vi "ReadPanelData.vi"(8 "error in (no error)":errorcluster, 11 "MAUI in":refnum<class "SMO.UI.MAUI.lvclass">) -> (0 "error out":errorcluster, 3 "MAUI out":refnum<class "SMO.UI.MAUI.lvclass">)   [LabVIEW 2019, in "SMO.UI.MAUI.lvclass"]
uses:
  SMO.UI.MAUI.lvclass
  Typedefs/PanelData.ctl
panel:
  in  "timeout in ms (-1)":i32
  out "last notification":T1[](array[typedef])
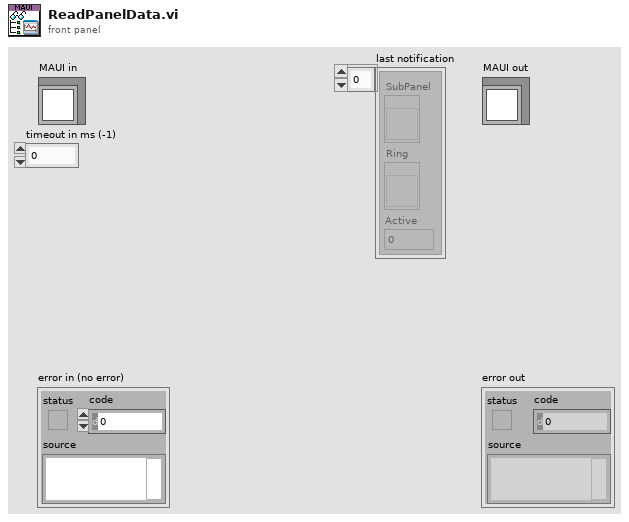
[diagram p1: front panel]
types:
  T1 = typedef "SMO.UI.MAUI.lvclass/PanelData.ctl" = cluster{"SubPanel":refnum<vi>, "Ring":refnum<vi>, "Active":i32}
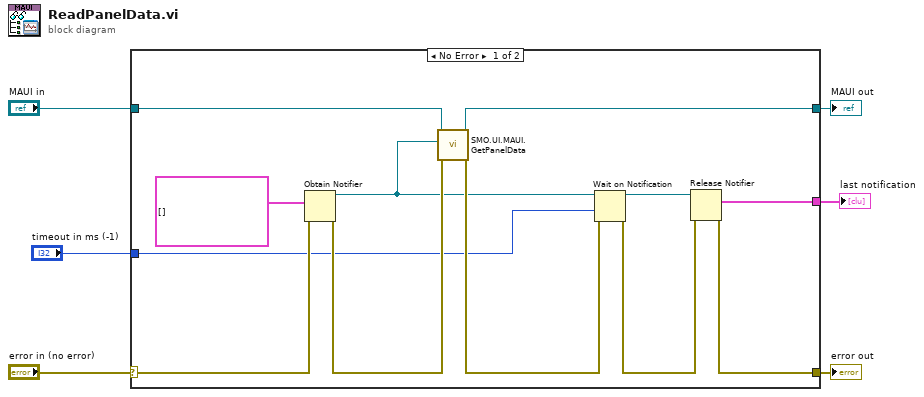
[diagram p0: block diagram]
diagram:
  n1 = case shown="No Error" "error in (no error)" {
    selector: "error in (no error)" -> [w18 w20]
    tunnel: [w14 w20] -> w5
    tunnel: [w8 w19] -> w3
    tunnel: "MAUI in" -> [w9 w19]
    tunnel: [w10 _] -> w2
    tunnel: "timeout in ms (-1)" -> [w7 _]
    frame No Error {
      n2 = Obtain Notifier(notification data type=T1[] [] ("Panel Data Array"), error in (no error)=w18) -> (notifier out=w11:refnum<notifier>, error out=w17:errorcluster)  [unwired: 2 in, 1 out]
      n3 = call "SMO.UI.MAUI.GetPanelData.vi"("error in (no error)"=w17, "GetPanelData"=w11, "MAUI"=w9) -> ("error out"=w16:errorcluster, "MAUI out"=w8:refnum<class "SMO.UI.MAUI.lvclass">)  [unwired: 7 in]
      n4 = Wait on Notification(notifier=w11, timeout in ms (-1)=w7, error in (no error)=w16) -> (notifier out=w12:refnum<notifier>, error out=w15:errorcluster)  [unwired: 1 in, 2 out]
      n5 = Release Notifier(notifier=w12, error in (no error)=w15) -> (last notification=w10:T1[], error out=w14:errorcluster)  [unwired: 1 in, 1 out]
    }
    frame Error {
    }
  }
  "error out" <- w5
  "MAUI out" <- w3
  "last notification" <- w2
